vi "Destroy to SSH.vi"(8 "Error In":errorcluster, 11 "Session":refnum<class "Session.lvclass">) -> (0 "Error Out":errorcluster, 3 "SSH":refnum<class "SSH.lvclass">)   [LabVIEW 2021, in "Field_RnD_Services_LIBSSH2_Toolkit.lvlib" / "Session.lvclass"]
doc: "Destroys this Session object and returns the SSH context used to originally create it."
uses:
  220524-VNA RP FLAT.llb/Session.lvclass
  220524-VNA RP FLAT.llb/SSH.lvclass
  220524-VNA RP FLAT.llb/Session.lvclass/Session.ctl
  220524-VNA RP FLAT.llb/Field_RnD_Services_LIBSSH2_Toolkit.lvlib
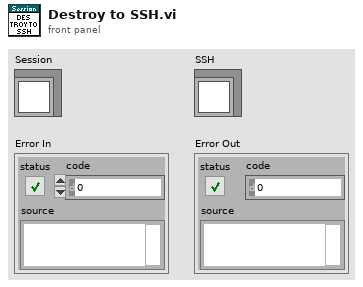
[diagram p1: front panel]
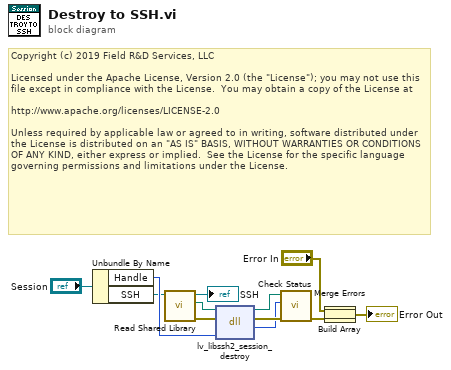
[diagram p0: block diagram]
diagram:
  # "Copyright (c) 2019 Field R&D Services, LLC\n\nLicensed under the Apache License, Version 2.0 (the \"License\"); you may not use this file except in compliance with the License.  You may obtain a copy of the License at\n\nhttp://www.apache.org/licenses/LICENSE-2.0\n\nUnless required by applicable law or agreed to in writing, software distributed under the License is distributed on an \"AS IS\" BASIS, WITHOUT WARRANTIES OR CONDITIONS OF ANY KIND, either express or implied.  See the License for the specific language governing permissions and limitations under the License."
  n1 = Unbundle By Name("Session") -> ("Handle"=w11:u64, "SSH"=w5:refnum<class "SSH.lvclass">)
  n2 = call "Read Shared Library.vi"("SSH In"=w5) -> ("Error Out"=w2:errorcluster, "libssh2lv Shared Library"=w3:path, "SSH Out"=→"SSH":refnum<class "SSH.lvclass">)  [unwired: 8 in]
  n3 = dll-call lib="libssh2lv.*" fn="lv_libssh2_session_destroy"(path in=w3, error in=w2, "handle"=w11) -> (path out=w8:path, error out=w9:errorcluster, "status"=w6:i32)  [unwired: 2 in]
  n4 = call "Check Status.vi"("Error In"=w9, "Status"=w6, "libssh2lv Shared Library In"=w8) -> ("Error Out"=w7:errorcluster)  [unwired: 7 in, 1 out]
  n5 = Build Array("Error In", w7) -> (w1:errorcluster[])
  n6 = Merge Errors(w1) -> (→"Error Out":errorcluster)
